vi "Launch Test Runner Actor.vi"(8 "error in (no error)":errorcluster, 10 "SequncePath":string, 11 "TestBench in":refnum<class "TestBench.lvclass">) -> (0 "error out":errorcluster, 3 "TestBench out":refnum<class "TestBench.lvclass">)   [LabVIEW 2019, in "TestBench.lvlib" / "TestBench.lvclass"]
uses:
  TestBench.lvclass
  C:/Program Files (x86)/National Instruments/LabVIEW 2019/vi.lib/ActorFramework/Actor/Actor.lvclass
  TestRunner/TestRunner/TestRunnerEvent.lvclass
  C:/Program Files (x86)/National Instruments/LabVIEW 2019/vi.lib/NI/Event Source Actor/Event Source/Event/Event.lvclass
  TestBench Messages/Write Execute Test VIs Msg/Write Execute Test VIs Msg.lvclass
  C:/Program Files (x86)/National Instruments/LabVIEW 2019/vi.lib/NI/Event Source Actor/Event Source/Event Source Messages/Event Generated Msg/Event Generated Msg.lvclass
  TestBench Messages/TestComplete Msg/TestComplete Msg.lvclass
  TestBench Messages/New Test Msg/New Test Msg.lvclass
  TestBench Messages/UpDataResult Msg/UpDataResult Msg.lvclass
  Assert/Assert/Assert Event.lvclass
  TestBench Messages/UploadSerialNumber Msg/UploadSerialNumber Msg.lvclass
  TestBench.lvclass/TestBench.ctl
  <vilib>/NI/Event Source Actor/Event Source/Event/Event.lvclass/Event.ctl
  TestEngine/TestEngine Messages/LunchTest Msg/LauncherTest Msg.lvclass/LauncherTest Msg.ctl
  <vilib>/ActorFramework/Message Enqueuer/Message Enqueuer.lvclass/Message Enqueuer.ctl
  <vilib>/ActorFramework/Actor/Actor.lvclass/Actor.ctl
  <vilib>/NI/Event Source Actor/Event Source/Event Source Messages/Register Msg/Register Msg.lvclass/Register Msg.ctl
  TestRunner/TestRunner Messages/Run Msg/Run Msg.lvclass/Run Msg.ctl
  32588125-fd70-4a76-8c39-565d81f41811.vi
  2f7d007b-58d7-4c28-bcf8-cd7960f4a7c9.vi
  <vilib>/ActorFramework/Message Enqueuer/Enqueue.vi
  <vilib>/ActorFramework/Message Enqueuer/Init from Existing Queue.vi
  TestRunner/TestRunner/TestRunner.lvclass
  Assert/Assert/Assert.lvclass
  TestEngine/TestEngine Messages/LunchTest Msg/LauncherTest Msg.lvclass
  C:/Program Files (x86)/National Instruments/LabVIEW 2019/vi.lib/ActorFramework/Message/Message.lvclass
  <vilib>/NI/Event Source Actor/Event Source/Event Source Messages/Register Msg/Register Msg.lvclass
  TestRunner/TestRunner Messages/Run Msg/Run Msg.lvclass
  <vilib>/ActorFramework/Message Priority Queue/Priority Enqueue.vi
  <vilib>/ActorFramework/Message Enqueuer/Message Enqueuer.lvclass
  <vilib>/ActorFramework/Actor/Actor.lvclass
  <vilib>/NI/Event Source Actor/Event Source/Event/Event.lvclass
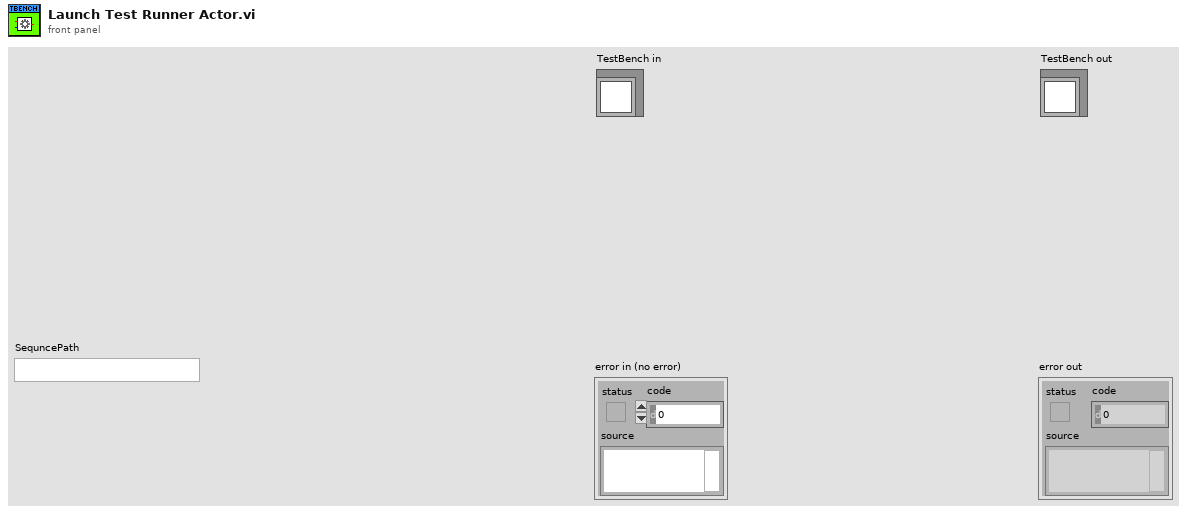
[diagram p1: front panel]
types:
  T1 = map{string, refnum<class "Message Enqueuer.lvclass">}
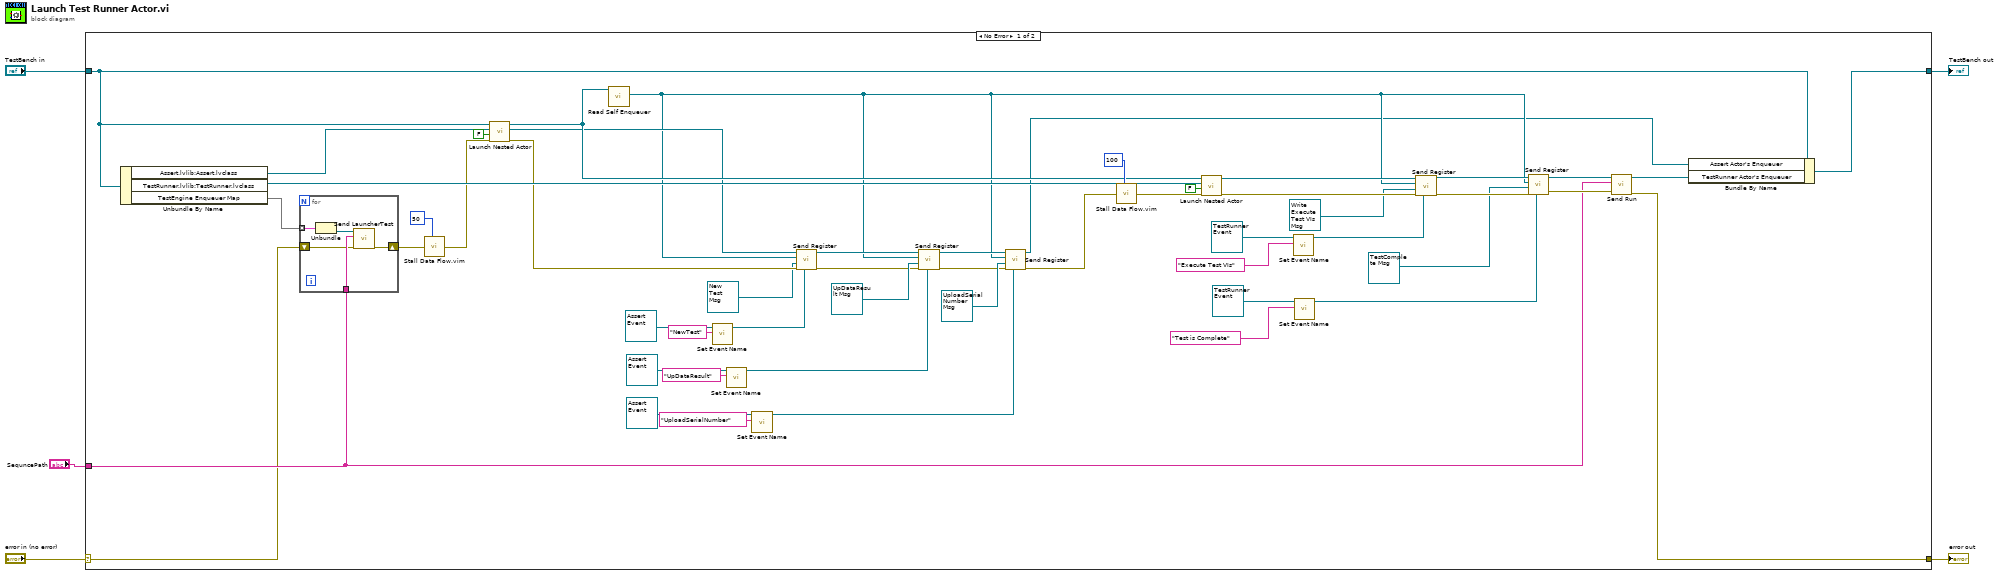
[diagram p0: block diagram]
diagram:
  n1 = case shown="No Error" "error in (no error)" {
    selector: "error in (no error)" -> [w31 w64]
    tunnel: [w35 w64] -> w4
    tunnel: [w36 w63] -> w2
    tunnel: "TestBench in" -> [w37 w63]
    tunnel: "SequncePath" -> [w33 _]
    frame No Error {
      n2 = Unbundle By Name(w37) -> ("Assert.lvlib:Assert.lvclass"=w42:refnum<class "Assert.lvclass">, "TestRunner.lvlib:TestRunner.lvclass"=w57:refnum<class "TestRunner.lvclass">, "TestEngine Enqueuer Map"=w34:T1)
      n3 = for {
        tunnel: w34 -> [w62] mode=indexing
        tunnel: w33 -> [w60]
        shift-right: [w59] -> w32
        shift-left: w31 -> [w58]
        n4 = Unbundle(w62) -> ("TestEngine Actor's Enqueuer"=w61:refnum<class "Message Enqueuer.lvclass">)  [unwired: 1 out]
        n5 = call "Send LauncherTest.vi"("error in (no error)"=w58, "SequncePath"=w60, "Message Enqueuer"=w61) -> ("error out"=w59:errorcluster)  [unwired: 7 in, 1 out]
      }
      n6 = call "Stall Data Flow.vim"("value in"=w32, "milliseconds to wait"=u32 50) -> ("value out"=w30:errorcluster)  [unwired: 1 out]
      n7 = call <vilib>:"Launch Nested Actor.vi"("error in (no error)"=w30, "Auto-stop? (T)"=FALSE, "Nested Actor"=w42, "Caller Actor in"=w37) -> ("error out"=w20:errorcluster, "Nested Actor's Enqueuer"=w23:refnum<class "Message Enqueuer.lvclass">, "Caller Actor out"=w38:refnum<class "TestBench.lvclass">)  [unwired: 5 in]
      n8 = call <vilib>:"Read Self Enqueuer.vi"("Actor"=w38) -> ("Self Enqueuer"=w8:refnum<class "Message Enqueuer.lvclass">)  [unwired: 10 in]
      n9 = call <vilib>:"Set Event Name.vi"("Name (Generic)"="NewTest", "Event In"=refnum<class "Assert Event.lvclass"> refnum ("Assert.lvlib:Assert Event.lvclass")) -> ("Event Out"=w25:refnum<class "Assert Event.lvclass">)  [unwired: 9 in]
      n10 = call <vilib>:"Set Event Name.vi"("Name (Generic)"="UpDataResult", "Event In"=refnum<class "Assert Event.lvclass"> refnum ("Assert.lvlib:Assert Event.lvclass")) -> ("Event Out"=w16:refnum<class "Assert Event.lvclass">)  [unwired: 9 in]
      n11 = call <vilib>:"Set Event Name.vi"("Name (Generic)"="UploadSerialNumber", "Event In"=refnum<class "Assert Event.lvclass"> refnum ("Assert.lvlib:Assert Event.lvclass")) -> ("Event Out"=w11:refnum<class "Assert Event.lvclass">)  [unwired: 9 in]
      n12 = call <vilib>:"Send Register.vi"("Event"=w25, "Error In"=w20, "Event Handler"=refnum<class "New Test Msg.lvclass"> refnum ("TestBench.lvlib:New Test Msg.lvclass"), "Registrant Address"=w8, "Event Source Address"=w23) -> ("Error Out"=w14:errorcluster, "Event Source Address Out"=w22:refnum<class "Message Enqueuer.lvclass">)  [unwired: 5 in]
      n13 = call <vilib>:"Send Register.vi"("Event"=w16, "Error In"=w14, "Event Handler"=refnum<class "UpDataResult Msg.lvclass"> refnum ("TestBench.lvlib:UpDataResult Msg.lvclass"), "Registrant Address"=w8, "Event Source Address"=w22) -> ("Error Out"=w9:errorcluster, "Event Source Address Out"=w21:refnum<class "Message Enqueuer.lvclass">)  [unwired: 5 in]
      n14 = call <vilib>:"Send Register.vi"("Event"=w11, "Error In"=w9, "Event Handler"=refnum<class "UploadSerialNumber Msg.lvclass"> refnum ("TestBench.lvlib:UploadSerialNumber Msg.lvclass"), "Registrant Address"=w8, "Event Source Address"=w21) -> ("Error Out"=w7:errorcluster, "Event Source Address Out"=w6:refnum<class "Message Enqueuer.lvclass">)  [unwired: 5 in]
      n15 = call "Stall Data Flow.vim"("value in"=w7, "milliseconds to wait"=u32 100) -> ("value out"=w41:errorcluster)  [unwired: 1 out]
      n16 = call <vilib>:"Launch Nested Actor.vi"("error in (no error)"=w41, "Auto-stop? (T)"=FALSE, "Nested Actor"=w57, "Caller Actor in"=w38) -> ("error out"=w46:errorcluster, "Nested Actor's Enqueuer"=w51:refnum<class "Message Enqueuer.lvclass">)  [unwired: 5 in, 1 out]
      n17 = call <vilib>:"Set Event Name.vi"("Name (Generic)"="Execute Test VIs", "Event In"=refnum<class "TestRunnerEvent.lvclass"> refnum ("UnitTestEngine.lvlib:TestRunnerEvent.lvclass")) -> ("Event Out"=w52:refnum<class "TestRunnerEvent.lvclass">)  [unwired: 9 in]
      n18 = call <vilib>:"Set Event Name.vi"("Name (Generic)"="Test is Complete", "Event In"=refnum<class "TestRunnerEvent.lvclass"> refnum ("UnitTestEngine.lvlib:TestRunnerEvent.lvclass")) -> ("Event Out"=w44:refnum<class "TestRunnerEvent.lvclass">)  [unwired: 9 in]
      n19 = call <vilib>:"Send Register.vi"("Event"=w52, "Error In"=w46, "Event Handler"=refnum<class "Write Execute Test VIs Msg.lvclass"> refnum ("TestBench.lvlib:Write Execute Test VIs Msg.lvclass"), "Registrant Address"=w8, "Event Source Address"=w51) -> ("Error Out"=w45:errorcluster, "Event Source Address Out"=w50:refnum<class "Message Enqueuer.lvclass">)  [unwired: 5 in]
      n20 = call <vilib>:"Send Register.vi"("Event"=w44, "Error In"=w45, "Event Handler"=refnum<class "TestComplete Msg.lvclass"> refnum ("TestBench.lvlib:TestComplete Msg.lvclass"), "Registrant Address"=w8, "Event Source Address"=w50) -> ("Error Out"=w43:errorcluster, "Event Source Address Out"=w49:refnum<class "Message Enqueuer.lvclass">)  [unwired: 5 in]
      n21 = call "Send Run.vi"("error in (no error)"=w43, "Libray Path"=w33, "Message Enqueuer"=w49) -> ("error out"=w35:errorcluster, "Message Enqueuer out"=w56:refnum<class "Message Enqueuer.lvclass">)  [unwired: 7 in]
      n22 = Bundle By Name(cluster=w37, "Assert Actor's Enqueuer"=w6, "TestRunner Actor's Enqueuer"=w56) -> (w36:refnum<class "TestBench.lvclass">)
    }
    frame Error {
    }
  }
  "error out" <- w4
  "TestBench out" <- w2
